vi "arm control.vi"(1 "State":T1, 2 "Z Axis (Tuning)":dbl) -> (0 "setpoint":dbl format="%.2f")   [LabVIEW 2013]
uses:
  typedefs/subStates.ctl
  typedefs/fg_typedef.ctl
panel:
  in  "2nd up setpoint":dbl format="%#_13g"
  in  "1st Up setpoint":dbl format="%#_13g"
  # "Things needing Tuning"
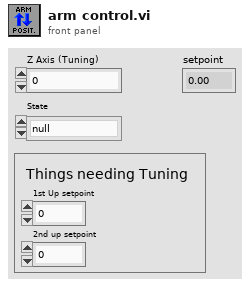
[diagram p1: front panel]
types:
  T1 = typedef "subStates.ctl" = enum16{"null", "wait", "driver control", "auto", "manual override", "hold position", "rotate", "pickup", "pass", "load", "goto shoot", "shoot", "end"}
  T2 = typedef "fg_typedef.ctl" = enum16{"Get", "Set"}
  T3 = typedef "WPI_DigitalInputDevRef.ctl" = cluster{"DevStatus":errorcluster, "DIO Channel":T4, "Digital Module":T5}
  T4 = typedef "FPGA_DIOChannel.ctl" = enum8{"DIO 1", "DIO 2", "DIO 3", "DIO 4", "DIO 5", "DIO 6", "DIO 7", "DIO 8", "DIO 9", "DIO 10", "DIO 11", "DIO 12", "DIO 13", "DIO 14", "Invalid"}
  T5 = typedef "FPGA_TypedefDigitalModule.ctl" = enum16{"Digital Module 1", "Digital Module 2"}
  T6 = typedef "WPI_EncoderDevRef.ctl" = cluster{"DevStatus":errorcluster, "EncoderIndex":T7, "CounterIndex":T8, "DistancePerCount":dbl, "Decoding Type":T9}
  T7 = typedef "FPGA_EncoderIdx.ctl" = enum8{"Enc 0", "Enc 1", "Enc 2", "Enc 3", "Invalid"}
  T8 = typedef "FPGA_CounterCtrSystemIndex.ctl" = enum8{"Ctr 0", "Ctr 1", "Ctr 2", "Ctr 3", "Ctr 4", "Ctr 5", "Ctr 6", "Ctr 7", "Invalid"}
  T9 = typedef "WPI_EncoderType.ctl" = enum16{"1x", "2x", "4x"}
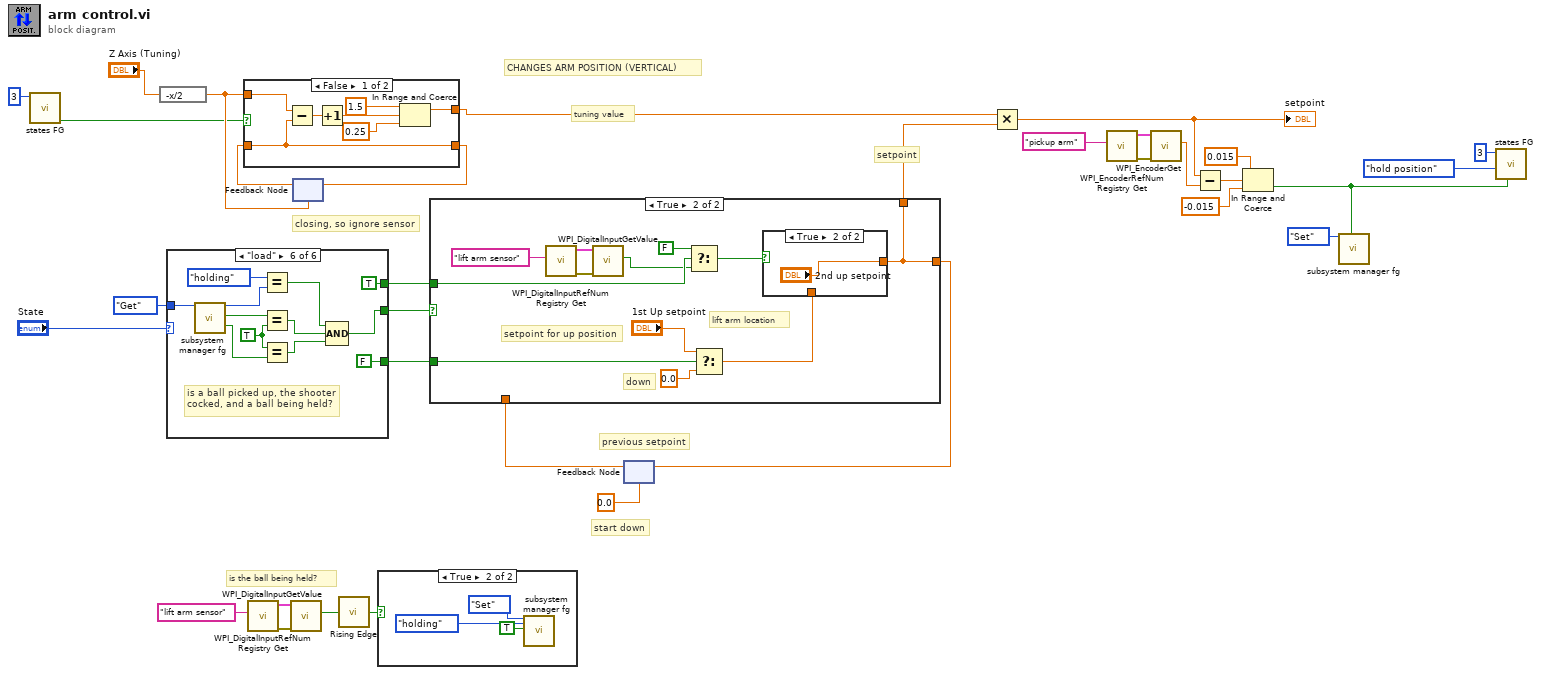
[diagram p0: block diagram]
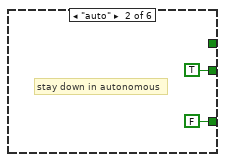
[diagram p6: hidden frame]
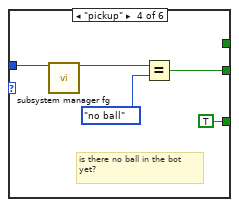
[diagram p8: hidden frame]
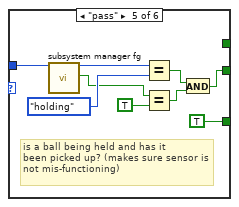
[diagram p9: hidden frame]
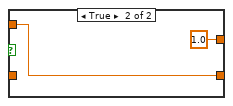
[diagram p10: hidden frame]
diagram:
  # "is the ball being held?"
  # "closing, so ignore sensor"
  # "start down"
  # "CHANGES ARM POSITION (VERTICAL)"
  # "previous setpoint"
  # "tuning value"
  # "setpoint"
  n1 = call "states FG.vi"("Loop ID"=3) -> ("first call?"=w22:bool)  [unwired: 7 in, 3 out]
  n2 = expression code="-x/2"("Z Axis (Tuning)") -> (w33:dbl)
  n3 = case shown="\"load\"" "State" {
    tunnel: fg_typedef."Get" ("Menu") -> [_ _ _ w40 w49 w60]
    tunnel: [_ TRUE _ w38 w42 w54] -> w18
    tunnel: [_ FALSE ("y") _ TRUE ("y") TRUE ("y") FALSE ("y")] -> w16
    tunnel: [_ _ _ _ _ TRUE ("y")] -> w6
    frame "driver control", Default {
      # "code does not run"
    }
    frame "auto" {
      # "stay down in autonomous"
    }
    frame "manual override" {
      # "code does not run"
    }
    frame "pickup" {
      # "is there no ball in the bot\nyet?"
      n4 = call "subsystem manager fg.vi"("Menu"=w40) -> ("Ball State Read"=w39:enum16{"no ball", "holding", "loaded"})  [unwired: 14 in, 4 out]
      n5 = Equal?(x=w39, y=enum16{"no ball", "holding", "loaded"}."no ball") -> (x = y?=w38:bool)
    }
    frame "pass" {
      # "is a ball being held and has it\nbeen picked up? (makes sure sensor is\nnot mis-functioning)"
      n6 = call "subsystem manager fg.vi"("Menu"=w49) -> ("Ball State Read"=w48:enum16{"no ball", "holding", "loaded"}, "Picked Up"=w46:bool)  [unwired: 14 in, 3 out]
      n7 = Equal?(x=w48, y=enum16{"no ball", "holding", "loaded"}."holding") -> (x = y?=w43:bool)
      n8 = Equal?(x=w46, y=TRUE) -> (x = y?=w44:bool)
      n9 = And(x=w43, y=w44) -> (x .and. y?=w42:bool)
    }
    frame "load" {
      w57 = TRUE ("y")
      # "is a ball picked up, the shooter\ncocked, and a ball being held?"
      n10 = call "subsystem manager fg.vi"("Menu"=w60) -> ("Ball State Read"=w53:enum16{"no ball", "holding", "loaded"}, "Picked Up"=w59:bool, "Shooter Cocked"=w58:bool)  [unwired: 14 in, 2 out]
      n11 = Equal?(x=enum16{"no ball", "holding", "loaded"}."holding", y=w53) -> (x = y?=w51:bool)
      n12 = Equal?(x=w59, y=w57) -> (x = y?=w56:bool)
      n13 = Equal?(x=w57, y=w58) -> (x = y?=w55:bool)
      n14 = Compound Arithmetic op=AND(w51, w56, w55) -> (w54:bool)
    }
  }
  n15 = call <vilib>:"WPI_DigitalInputRefNum Registry Get.vi"("refnum name"="lift arm sensor") -> ("error out"=w1:errorcluster, "DigitalInputDevRef"=w2:T3)  [unwired: 9 in]
  n16 = call <vilib>:"WPI_DigitalInputGetValue.vi"("error in (no error)"=w1, "DigitalInputDevRef"=w2) -> ("Value"=w4:bool)  [unwired: 7 in, 2 out]
  n17 = feedback #1(w33) -> (w31:dbl)
  n18 = case shown="False" w22 {
    tunnel: w33 -> [w68 w70]
    tunnel: [w67 w70] -> w30
    tunnel: w31 -> [w67 _]
    tunnel: [w64 1.0 ("upper limit")] -> w17
    frame False {
      n19 = Subtract(x=w68, y=w67) -> (x-y=w63:dbl)
      n20 = Increment(x=w63) -> (x+1=w62:dbl)
      n21 = In Range and Coerce(upper limit=1.5, x=w62, lower limit=0.25) -> (coerced(x)=w64:dbl)  [unwired: 1 out]
    }
    frame True {
    }
  }
  n22 = feedback-in #1(w30) -> ()
  n23 = call "Rising Edge.vi"("Input"=w4) -> ("Rising Edge"=w5:bool)
  n24 = case shown="True" w5 {
    frame False {
    }
    frame True {
      n25 = call "subsystem manager fg.vi"("Menu"=fg_typedef."Set", "Ball State Write"=enum16{"no ball", "holding", "loaded"}."holding", "Picked Up"=TRUE) -> ()  [unwired: 12 in, 5 out]
    }
  }
  n26 = feedback #2(0.0 ("x")) -> (w8:dbl)
  n27 = case shown="True" w18 {
    tunnel: w16 -> [_ w84]
    tunnel: [w74 w79] -> w10
    tunnel: [w74 w79] -> w9
    tunnel: w8 -> [w74 _]
    tunnel: w6 -> [_ w77]
    frame False {
      # "stay at previous location"
      # "the robot is not ready to run this code yet"
    }
    frame True {
      # "lift arm location"
      # "down"
      # "setpoint for up position"
      n28 = call <vilib>:"WPI_DigitalInputRefNum Registry Get.vi"("refnum name"="lift arm sensor") -> ("error out"=w81:errorcluster, "DigitalInputDevRef"=w82:T3)  [unwired: 9 in]
      n29 = call <vilib>:"WPI_DigitalInputGetValue.vi"("error in (no error)"=w81, "DigitalInputDevRef"=w82) -> ("Value"=w76:bool)  [unwired: 7 in, 2 out]
      n30 = Select(t=FALSE, s=w77, f=w76) -> (s? t:f=w78:bool)
      n31 = Select(t="1st Up setpoint", s=w84, f=0.0 ("x")) -> (s? t:f=w80:dbl)
      n32 = case shown="True" w78 {
        tunnel: w80 -> [w87 _]
        tunnel: [w87 "2nd up setpoint"] -> w79
        frame False {
        }
        frame True {
        }
      }
    }
  }
  n33 = feedback-in #2(w9) -> ()
  n34 = Multiply(x=w17, y=w10) -> (x*y=w15:dbl)
  "setpoint" <- w15
  n35 = call <vilib>:"WPI_EncoderRefNum Registry Get.vi"("refnum name"="pickup arm") -> ("error out"=w23:errorcluster, "EncoderDevRef"=w24:T6)  [unwired: 9 in]
  n36 = call <vilib>:"WPI_EncoderGet.vi"("error in (no error)"=w23, "EncoderDevRef"=w24) -> ("Distance"=w29:dbl)  [unwired: 4 in, 5 out]
  n37 = Subtract(x=w15, y=w29) -> (x-y=w26:dbl)
  n38 = In Range and Coerce(upper limit=0.015, x=w26, lower limit=-0.015) -> (In Range?=w12:bool)  [unwired: 1 out]
  n39 = call "subsystem manager fg.vi"("Menu"=fg_typedef."Set", "Arm Ready"=w12) -> ()  [unwired: 13 in, 5 out]
  n40 = call "states FG.vi"("exit in"=w12, "subState in"=subStates."hold position", "Loop ID"=3) -> ()  [unwired: 5 in, 4 out]
